vi "time3.vi"() -> ()   [LabVIEW 2020]
panel:
  out "time 3":T1
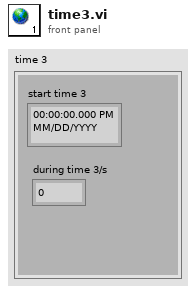
[diagram p1: front panel]
types:
  T1 = cluster{"start time 3":timestamp, "during time 3/s":dbl}
diagram:
